vi "Execute.vi"(8 "error in (no error)":errorcluster, 10 "Abstract Consumer in":refnum<class "Abstract Consumer.lvclass">, 11 "Log Message in":refnum<class "Manage File Request.lvclass">) -> (0 "error out":errorcluster, 1 "Abstract Response out":refnum<class "Abstract Response Message.lvclass">, 2 "Abstract Consumer out":refnum<class "Abstract Consumer.lvclass">, 3 "Log Message out":refnum<class "Manage File Request.lvclass">, 4 "Stop?":bool)   [LabVIEW 2020, in "AIM ARINC 664 Engine.lvlib" / "Implementation.lvlib" / "Frame Logging.lvlib" / "Manage File Request.lvclass"]
uses:
  Manage File Request.lvclass
  <vilib>/NI/VeriStand Custom Device Messaging/Consumer/Abstract Consumer/Abstract Consumer.lvclass
  <vilib>/NI/VeriStand Custom Device Messaging/Message/Abstract Response Message/Abstract Response Message.lvclass
  Manage File Response/Manage File Response.lvclass
  C:/Program Files (x86)/National Instruments/LabVIEW 2020/vi.lib/NI/VeriStand Custom Device Messaging/Message/Abstract Response Message/Abstract Response Message.lvclass
  Manage File Request.lvclass/Manage File Request.ctl
  Manage File Response/Manage File Response.lvclass/Manage File Response.ctl
  Read Logger.vi
  Read Log File Directory.vi
  Read Base name.vi
  Read Timestamp.vi
  Manage File Response/Write current filename.vi
  Manage File Response/Write log in progress.vi
  Logger Interface/Logger Interface.lvclass
  Frame Logging.lvlib
  C:/Program Files (x86)/National Instruments/LabVIEW 2020/vi.lib/NI/VeriStand Custom Device Messaging/Message/Abstract Message/Abstract Message.lvclass
  C:/Users/Administrator/Desktop/GIT/niveristand-aim-arinc664-custom-device/Source/Custom Device Support/Engine/Implementation/Logging/Frame Logging/Manage File Response/Manage File Response.lvclass
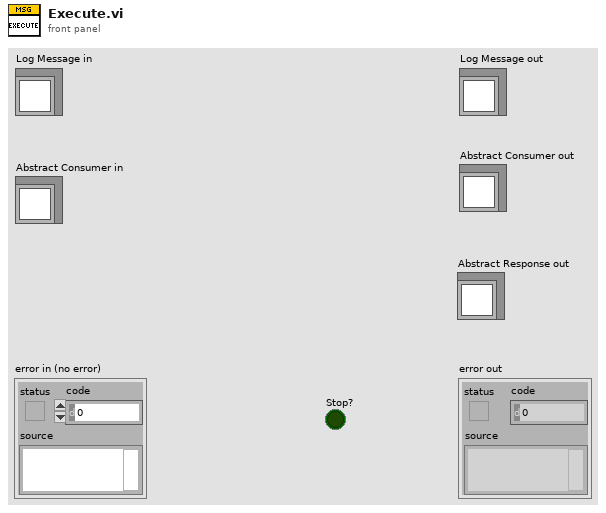
[diagram p1: front panel]
types:
  T1 = typedef "AIM ARINC 664 Engine.lvlib/Implementation.lvlib/Frame Logging.lvlib/Logger Data Reference.ctl" = refnum<data-value>
  T2 = typedef "AIM ARINC 664 Engine.lvlib/Implementation.lvlib/Monitor Execution Unit.lvclass/loggingThreshold_types.ctl" = cluster{"threashold_MB":dbl, "duration_sec":dbl, "DiskSpaceThPerc":dbl, "checkDiskSpace":bool, "segmentFiles":bool, "Segment Files By":T3}
  T3 = typedef "FileSegmentType.ctl" = enum16{"Time", "Size"}
  T4 = cluster{"Logger Interface.lvclass":refnum<class "Logger Interface.lvclass">}
  T5 = enum16{"no action", "close file", "segment file"}
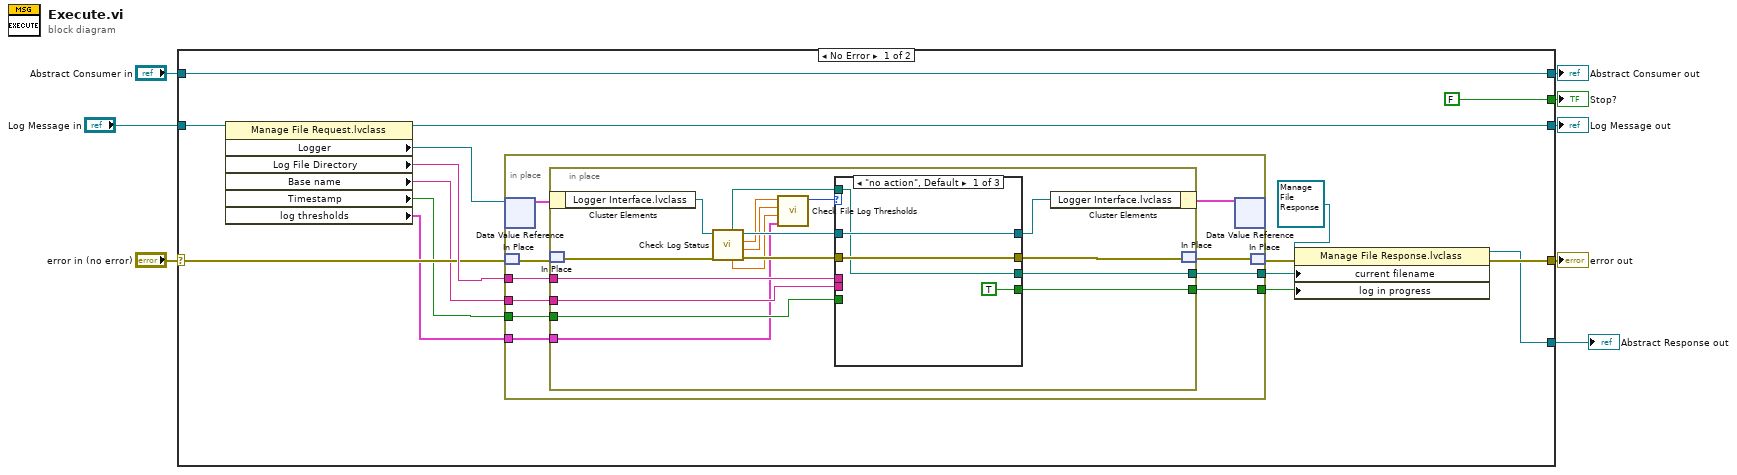
[diagram p0: block diagram]
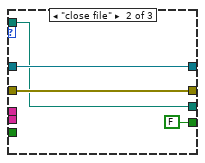
[diagram p2: hidden frame]
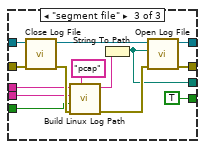
[diagram p3: hidden frame]
diagram:
  n1 = case shown="No Error" "error in (no error)" {
    selector: "error in (no error)" -> [w19 w76]
    tunnel: [w14 w76] -> w7
    tunnel: [w18 w75] -> w6
    tunnel: "Log Message in" -> [w22 w75]
    tunnel: [w23 w74] -> w4
    tunnel: "Abstract Consumer in" -> [w23 w74]
    tunnel: [FALSE ("Stop?") _] -> w2
    tunnel: [w13 _] -> w1
    frame No Error {
      n2 = property class="Manage File Request.lvclass"(reference=w22) -> (reference out=w18:refnum<class "Manage File Request.lvclass">, "Logger"=w21:T1, "Log File Directory"=w20:string, "Base name"=w17:string, "Timestamp"=w16:bool, "log thresholds"=w9:T2)  [unwired: 1 in, 1 out]
      n3 = in-place {
        in-place-border: w20 -> [w30]
        in-place-border: w17 -> [w29]
        in-place-border: w16 -> [w28]
        in-place-border: [w27] -> w11
        in-place-border: [w26] -> w10
        in-place-border: w9 -> [w25]
        n4 = in-place-dvr #1(w21) -> (w34:T4)  [unwired: 1 out]
        n5 = in-place-match #2(w19) -> (w33:errorcluster)
        n6 = in-place {
          in-place-border: w30 -> [w46]
          in-place-border: w29 -> [w45]
          in-place-border: w28 -> [w44]
          in-place-border: [w43] -> w27
          in-place-border: [w37] -> w26
          in-place-border: w25 -> [w35]
          n7 = in-place-cluster #3(w34) -> ("Logger Interface.lvclass"=w51:refnum<class "Logger Interface.lvclass">)
          n8 = in-place-match #4(w33) -> (w50:errorcluster)
          n9 = call-dynamic "Check Log Status.vi"("error in"=w50, "Logger Interface in"=w51) -> ("error out"=w42:errorcluster, "Log duration sec"=w40:dbl, "Log file Size MB"=w41:dbl, "Logger Interface out"=w48:refnum<class "Logger Interface.lvclass">, "Hard Drive Space Used (%)"=w39:dbl, "current filename"=w36:path)  [unwired: 4 in]
          n10 = call "Check File Log Thresholds.vi"("log thresholds"=w35, "Hard Drive Space Used (%)"=w39, "Log duration sec"=w40, "Log file Size MB"=w41) -> ("action"=w38:T5)  [unwired: 7 in]
          n11 = case shown="\"no action\", Default" w38 {
            tunnel: w48 -> [w55 w59 w73]
            tunnel: w42 -> [w54 w58 w71]
            tunnel: [w54 w58 w70] -> w47
            tunnel: [w55 w59 w69] -> w49
            tunnel: w46 -> [_ _ w64]
            tunnel: w45 -> [_ _ w63]
            tunnel: w44 -> [_ _ w62]
            tunnel: [w52 w56 w61] -> w43
            tunnel: [TRUE ("log in progress") FALSE ("log in progress") TRUE ("log in progress")] -> w37
            tunnel: w36 -> [w52 w56 _]
            frame "no action", Default {
            }
            frame "close file" {
            }
            frame "segment file" {
              n12 = call-dynamic "Close Log File.vi"("error in (no error)"=w71, "Logger Interface in"=w73) -> ("error out"=w67:errorcluster, "Logger Interface out"=w72:refnum<class "Logger Interface.lvclass">)  [unwired: 8 in]
              n13 = call "Build Linux Log Path.vi"("Extension"="pcap", "error in (no error)"=w67, "Timestamp"=w62, "Name"=w63, "Log File Directory"=w64) -> ("error out"=w66:errorcluster, "Log File Path"=w65:string)  [unwired: 5 in]
              n14 = String To Path(string=w65) -> (path=w61:path)
              n15 = call-dynamic "Open Log File.vi"("error in (no error)"=w66, "Path"=w61, "Logger Interface in"=w72) -> ("error out"=w70:errorcluster, "Logger Interface out"=w69:refnum<class "Logger Interface.lvclass">)  [unwired: 7 in]
            }
          }
          n16 = in-place-cluster #3("Logger Interface.lvclass"=w49) -> (w32:T4)
          n17 = in-place-match #4(w47) -> (w31:errorcluster)
        }
        n18 = in-place-dvr #1(w32) -> ()  [unwired: 2 out]
        n19 = in-place-match #2(w31) -> (w15:errorcluster)
      }
      n20 = property class="Manage File Response.lvclass"(reference=refnum<class "Manage File Response.lvclass"> refnum ("Communication Bus Template Interfaces:Implementation.lvlib:Frame Logging.lvlib:Manage File Response.lvclass"), error in=w15, "current filename"=w11, "log in progress"=w10) -> (reference out=w13:refnum<class "Manage File Response.lvclass">, error out=w14:errorcluster)
    }
    frame Error {
    }
  }
  "error out" <- w7
  "Log Message out" <- w6
  "Abstract Consumer out" <- w4
  "Stop?" <- w2
  "Abstract Response out" <- w1
